vi "7.5 Hz Parker MagnePump Head-Flow Curves.vi"() -> (1 "speed / Hz":dbl[](array[numeric]), 2 "head / ft":dbl[](array[numeric]), 3 "flow / gpm":dbl[](array[numeric]))   [LabVIEW 2020]
uses:
  <vilib>/Utility/file.llb/Write Delimited Spreadsheet (DBL).vi
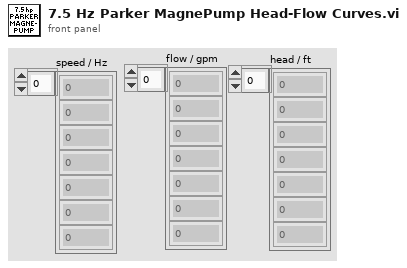
[diagram p1: front panel]
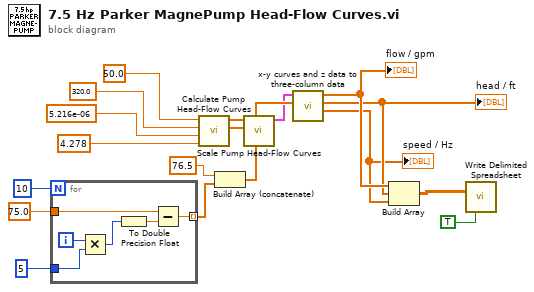
[diagram p0: block diagram]
diagram:
  n1 = for {
    N: 10 -> [_]
    tunnel: 75.0 -> [w21]
    tunnel: 5 -> [w23]
    tunnel: [w19] -> w16 mode=indexing
    i -> [w24]
    n2 = Multiply(x=w24, y=w23) -> (x*y=w22:i32)
    n3 = To Double Precision Float(number=w22) -> (double precision float=w20:dbl)
    n4 = Subtract(x=w21, y=w20) -> (x-y=w19:dbl)
  }
  n5 = call "Calculate Pump Head-Flow Curves.vi"("n"=4.278, "A"=5.216e-06, "Shut-off head"=320.0, "Run-out flow"=50.0) -> ("head"=w11:dbl[], "flow"=w10:dbl[])  [unwired: 6 in]
  n6 = Build Array (concatenate)(76.5, w16) -> (w18:dbl[])
  n7 = call "Scale Pump Head-Flow Curves.vi"("speeds"=w18, "head"=w11, "flow"=w10) -> ("head-flow curves"=w17:cluster{dbl[], dbl[]}[])  [unwired: 8 in]
  n8 = call "x-y curves and z data to three-column data.vi"("z label values"=w18, "x-y curves"=w17) -> ("z"=w3:dbl[], "y"=w4:dbl[], "x"=w5:dbl[])  [unwired: 7 in]
  "head / ft" <- w4
  "flow / gpm" <- w5
  "speed / Hz" <- w3
  n9 = Build Array(w5, w4, w3) -> (w2:dbl[][])
  n10 = call-poly <vilib>:"Write Delimited Spreadsheet.vi"("2D data"=w2, "transpose? (no:F)"=TRUE) -> ()  [unwired: 12 in, 2 out]
